vi "Image Acquisition Settings FG.vi"(8 "error in (no error)":errorcluster, 10 "Acquisition Settings In":T2={"Image Width"=2040, "Image Height"=1088, "Frames To Acquire"=0, "Signal Mapping"=enum."Basler 10-tap", "DMA Buffer Size\n(In Images)"=64} {"Image Height" max=65535; "Image Width" max=65535 step=40}, 11 "Operation":T1) -> (0 "error out":errorcluster, 2 "Acquisition Settings Out":T2={"Image Width"=2040, "Image Height"=1088, "Frames To Acquire"=0, "Signal Mapping"=enum."Basler 10-tap", "DMA Buffer Size\n(In Images)"=64} {"Image Height" max=65535; "Image Width" max=65535 step=40})   [LabVIEW 2013]
uses:
  Acquisition Settings Cluster.ctl
  Image Acquisition Settings FG Enum.ctl
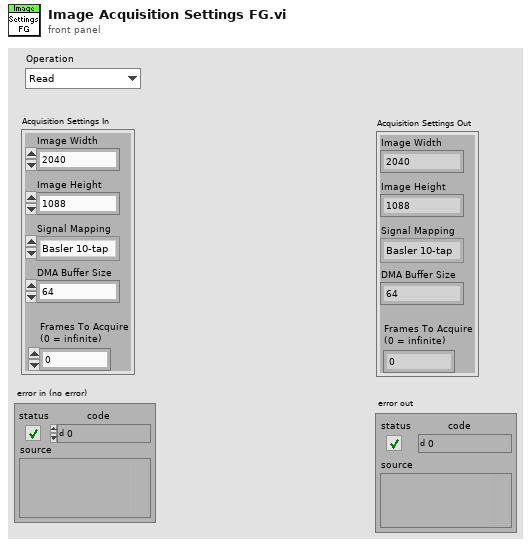
[diagram p1: front panel]
types:
  T1 = typedef "Image Acquisition Settings FG Enum.ctl" = enum16{"Read", "Write"}
  T2 = typedef "Acquisition Settings Cluster.ctl" = cluster{"Image Width":u32, "Image Height":u32, "Frames To Acquire":u32, "Signal Mapping":enum8{"Standard", "Basler 10-tap", "Vosskühler 10-tap"}, "DMA Buffer Size\n(In Images)":u32}
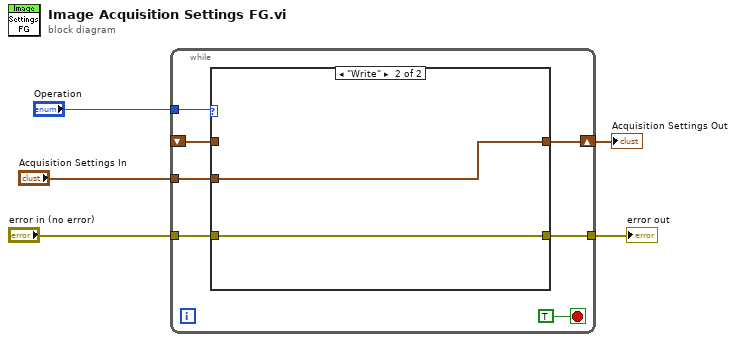
[diagram p0: block diagram]
diagram:
  n1 = while {
    tunnel: "Operation" -> [w11]
    tunnel: "Acquisition Settings In" -> [w10]
    shift-right: [w9] -> w3
    shift-left: _ -> [w8]
    tunnel: [w7] -> w2
    tunnel: "error in (no error)" -> [w6]
    stop <- TRUE stop-if-true
    n2 = case shown="\"Write\"" w11 {
      tunnel: w10 -> [_ w16]
      tunnel: [w14 w16] -> w9
      tunnel: w8 -> [w14 _]
      tunnel: [w13 w15] -> w7
      tunnel: w6 -> [w13 w15]
      frame "Read" {
      }
      frame "Write" {
      }
    }
  }
  "Acquisition Settings Out" <- w3
  "error out" <- w2
